vi "saveDAta.vi"(8 "error in (no error)":errorcluster, 10 "Numeric":dbl, 11 "Loggin in":refnum<class "Loggin.lvclass">) -> (0 "error out":errorcluster, 3 "Loggin out":refnum<class "Loggin.lvclass">)   [LabVIEW 2020, in "Loggin.lvlib" / "Loggin.lvclass"]
uses:
  Loggin.lvclass
  Loggin.lvclass/Loggin.ctl
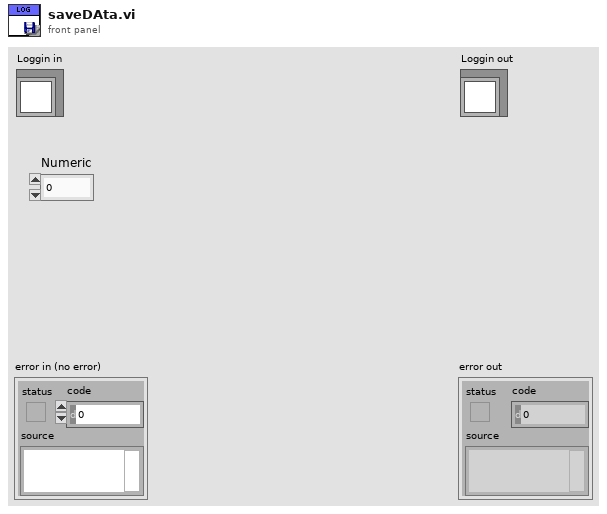
[diagram p1: front panel]
types:
  T1 = enum16{"open", "replace", "create", "open or create", "replace or create", "replace or create with confirmation"}
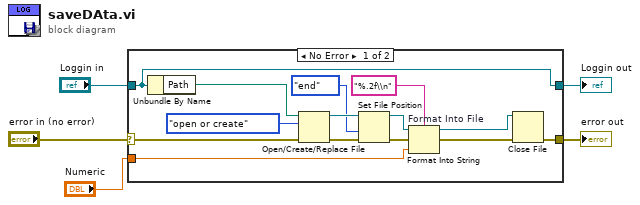
[diagram p0: block diagram]
diagram:
  n1 = case shown="No Error" "error in (no error)" {
    selector: "error in (no error)" -> [w16 w21]
    tunnel: [w14 w21] -> w4
    tunnel: [w19 w20] -> w2
    tunnel: "Loggin in" -> [w19 w20]
    tunnel: "Numeric" -> [w6 _]
    frame No Error {
      n2 = Unbundle By Name(w19) -> ("Path"=w18:path)
      n3 = Open/Create/Replace File(file path (use dialog)=w18, error in=w16, operation (0:open)=T1."open or create") -> (refnum out=w13:refnum<file>, error out=w15:errorcluster)  [unwired: 3 in, 1 out]
      n4 = Set File Position(refnum=w13, from (0:start)=enum16{"start", "end", "current"}."end", error in=w15) -> (refnum out=w10:refnum<file>, error out=w12:errorcluster)  [unwired: 1 in]
      n5 = Format Into String "Format Into File"(format string="%.2f\\n", initial string=w10, error in=w12, w6) -> (resulting string=w9:refnum<file>, error out=w11:errorcluster)
      n6 = Close File(refnum=w9, error in=w11) -> (error out=w14:errorcluster)  [unwired: 1 out]
    }
    frame Error {
    }
  }
  "error out" <- w4
  "Loggin out" <- w2
